vi "BUILD_install and upload core.vi"(9 "LabVIEW Version":string, 10 "Repository Name":string, 11 "appended path":path) -> (0 "error out":errorcluster)   [LabVIEW 2013]
uses:
  <vilib>/JKI/VIPM API/VIPM API_vipm_api.lvlib
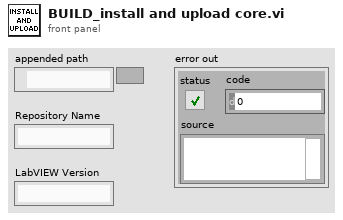
[diagram p1: front panel]
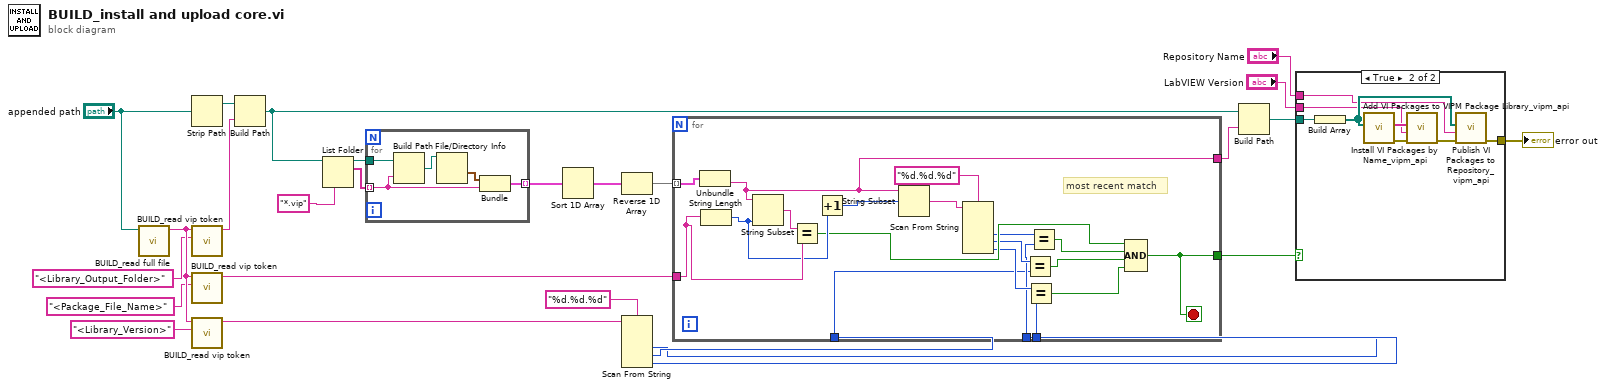
[diagram p0: block diagram]
diagram:
  n1 = call "BUILD_read full file.vi"("vip file"="appended path") -> ("data"=w22:string)  [unwired: 9 in, 1 out]
  n2 = Strip Path(path="appended path") -> (stripped path=w26:path)  [unwired: 1 out]
  n3 = call "BUILD_read vip token.vi"("regular expression"="<Library_Output_Folder>", "data"=w22) -> ("trimmed string"=w16:string)  [unwired: 9 in]
  n4 = call "BUILD_read vip token.vi"("regular expression"="<Package_File_Name>", "data"=w22) -> ("trimmed string"=w20:string)  [unwired: 9 in]
  n5 = call "BUILD_read vip token.vi"("regular expression"="<Library_Version>", "data"=w22) -> ("trimmed string"=w18:string)  [unwired: 9 in]
  n6 = Build Path(base path=w26, name or relative path=w16) -> (appended path=w12:path)
  n7 = List Folder(path=w12, pattern="*.vip") -> (path out=w2:path, filenames=w3:string[])  [unwired: 2 in, 2 out]
  n8 = for {
    tunnel: w2 -> [w31]
    tunnel: w3 -> [w28] mode=indexing
    tunnel: [w27] -> w4 mode=indexing
    n9 = Build Path(base path=w31, name or relative path=w28) -> (appended path=w30:path)
    n10 = File/Directory Info(path=w30) -> (last mod=w29:timestamp)  [unwired: 1 in, 6 out]
    n11 = Bundle("last mod"=w29, w28) -> (w27:cluster{"last mod":timestamp, string})  [unwired: 1 in]
  }
  n12 = Sort 1D Array(array=w4) -> (sorted array=w5:cluster{"last mod":timestamp, string}[])
  n13 = Reverse 1D Array(array=w5) -> (reversed array=w6:cluster{"last mod":timestamp, string}[])
  n14 = Scan From String(format string="%d.%d.%d", input string=w18) -> (output 1=w8:i32, output 2=w9:i32, output 3=w10:i32)  [unwired: 5 in, 3 out]
  n15 = for {
    tunnel: w6 -> [w50] mode=indexing
    tunnel: w20 -> [w48]
    tunnel: w8 -> [w36]
    tunnel: w9 -> [w35]
    tunnel: w10 -> [w34]
    tunnel: [w33] -> w11
    tunnel: [w32] -> w13
    stop <- w32 stop-if-true
    # "most recent match"
    n16 = Unbundle(w50) -> (w33:string)  [unwired: 1 out]
    n17 = String Length(string=w48) -> (length=w46:i32)
    n18 = String Subset(string=w33, length (rest)=w46) -> (substring=w49:string)  [unwired: 1 in]
    n19 = Equal?(x=w49, y=w48) -> (x = y?=w43:bool)
    n20 = Increment(x=w46) -> (x+1=w47:i32)
    n21 = String Subset(string=w33, offset (0)=w47) -> (substring=w45:string)  [unwired: 1 in]
    n22 = Scan From String(format string="%d.%d.%d", input string=w45) -> (output 1=w39:i32, output 2=w38:i32, output 3=w37:i32)  [unwired: 5 in, 3 out]
    n23 = Equal?(x=w38, y=w35) -> (x = y?=w41:bool)
    n24 = Equal?(x=w37, y=w34) -> (x = y?=w40:bool)
    n25 = Equal?(x=w39, y=w36) -> (x = y?=w42:bool)
    n26 = Compound Arithmetic op=AND(w43, w42, w41, w40) -> (w32:bool)
  }
  n27 = Build Path(base path=w12, name or relative path=w11) -> (appended path=w14:path)
  n28 = case shown="True" w13 {
    tunnel: w14 -> [_ w58]
    tunnel: [_ w53] -> w15
    tunnel: "LabVIEW Version" -> [_ w52]
    tunnel: "Repository Name" -> [_ w51]
    frame False {
    }
    frame True {
      n29 = Build Array(w58) -> (w57:path[])
      n30 = call <vilib>:"Add VI Packages to VIPM Package Library_vipm_api.vi"("Packages to add to VIPM Library (vipc,vip,ogp)"=w57) -> ("error out"=w56:errorcluster, "Package Names Added"=w55:string[])  [unwired: 9 in]
      n31 = call <vilib>:"Install VI Packages by Name_vipm_api.vi"("error in (no error)"=w56, "LabVIEW Version"=w52, "Package Names to Install []"=w55) -> ("error out"=w54:errorcluster)  [unwired: 8 in]
      n32 = call <vilib>:"Publish VI Packages to Repository_vipm_api.vi"("error in (no error)"=w54, "Repository Name"=w51, "Packages to publish to Repository Library (vip,ogp)"=w57) -> ("error out"=w53:errorcluster)  [unwired: 7 in, 1 out]
    }
  }
  "error out" <- w15
